vi "Login.vi"(8 "error in (no error)":errorcluster) -> (0 "error out":errorcluster)   [LabVIEW 2017]
uses:
  <vilib>/Utility/error.llb/DialogType.ctl
  Control/Login Authority CSV FGV Command.ctl
  Global/Login Details.vi
  Global/Global 1.vi
panel:
  in  "CANCEL":bool
  in  "LOGIN":bool
  in  "PASSWORD":string
  in  "USER NAME":string(combo)
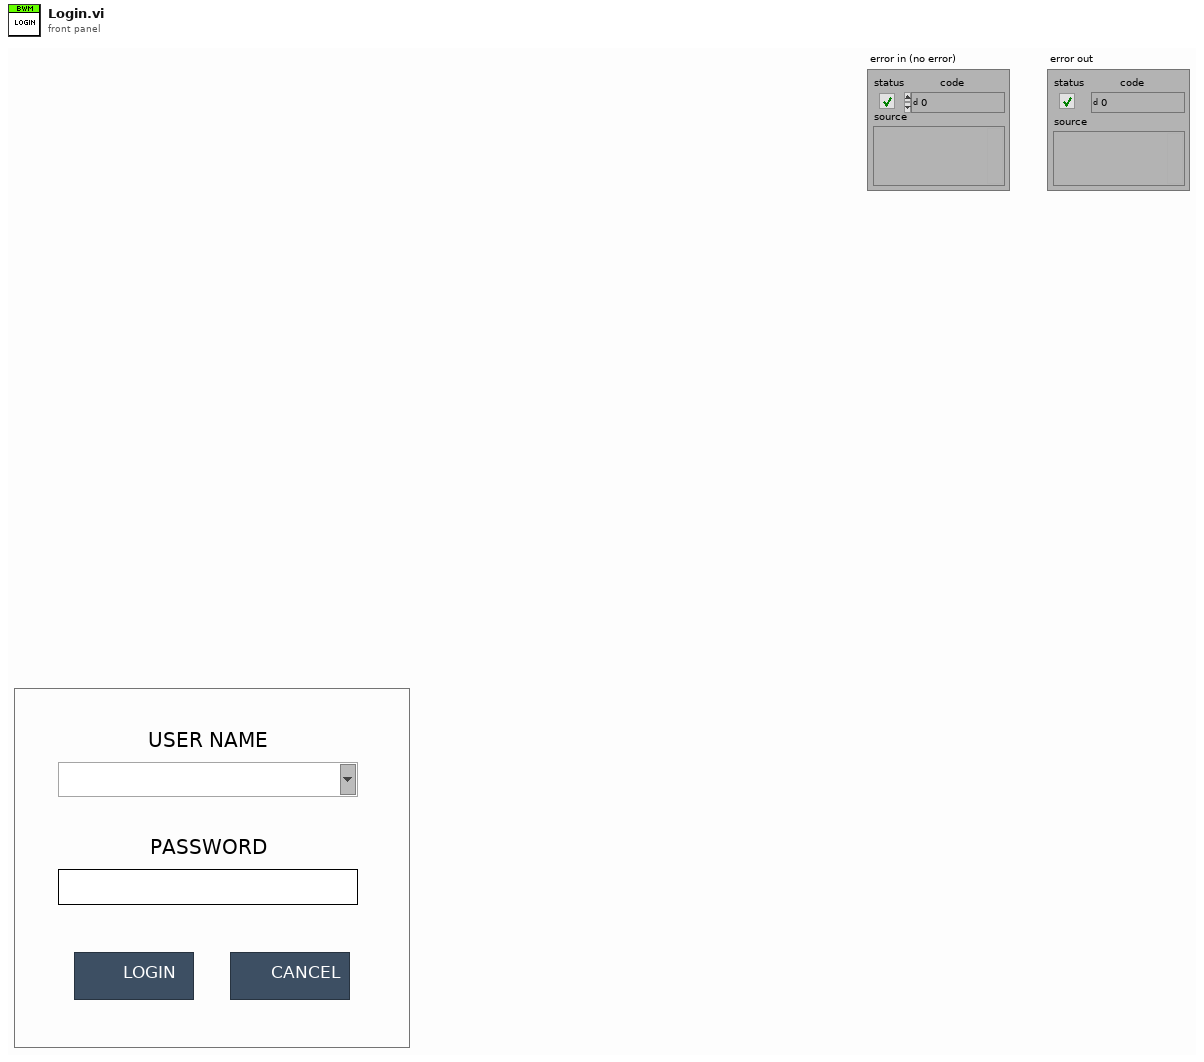
[diagram p1: front panel]
types:
  T1 = typedef "Login Authority CSV FGV Command.ctl" = enum16{"Init", "Save", "Read", "Get Data", "Delete"}
  T2 = typedef "DialogType.ctl" = u16
  T3 = enum32{"invalid app kind", "Development System", "Run Time System", "Student Edition", "Embedded LabVIEW", "Evaluation", "Custom"}
  T4 = cluster{"SCREEN 1":bool, "SCREEN 2":bool, "SCREEN 3":bool, "SCREEN 4":bool, "SCREEN 5":bool, "SCREEN 6":bool, "SCREEN 7":bool, "SCREEN 8":bool, "SCREEN 9":bool, "SCREEN 10":bool, "SCREEN 11":bool, "SCREEN 12":bool, "SCREEN 13":bool, "SCREEN 14":bool, "SCREEN 15":bool, "SCREEN 16":bool, "SCREEN 17":bool, "SCREEN 18":bool, "SCREEN 19":bool, "SCREEN 20":bool}
  T5 = cluster{"USERNAME":string, "AUTHORITY":string, "PASSWORD":string, "RE-ENTER PASSWORD":string}
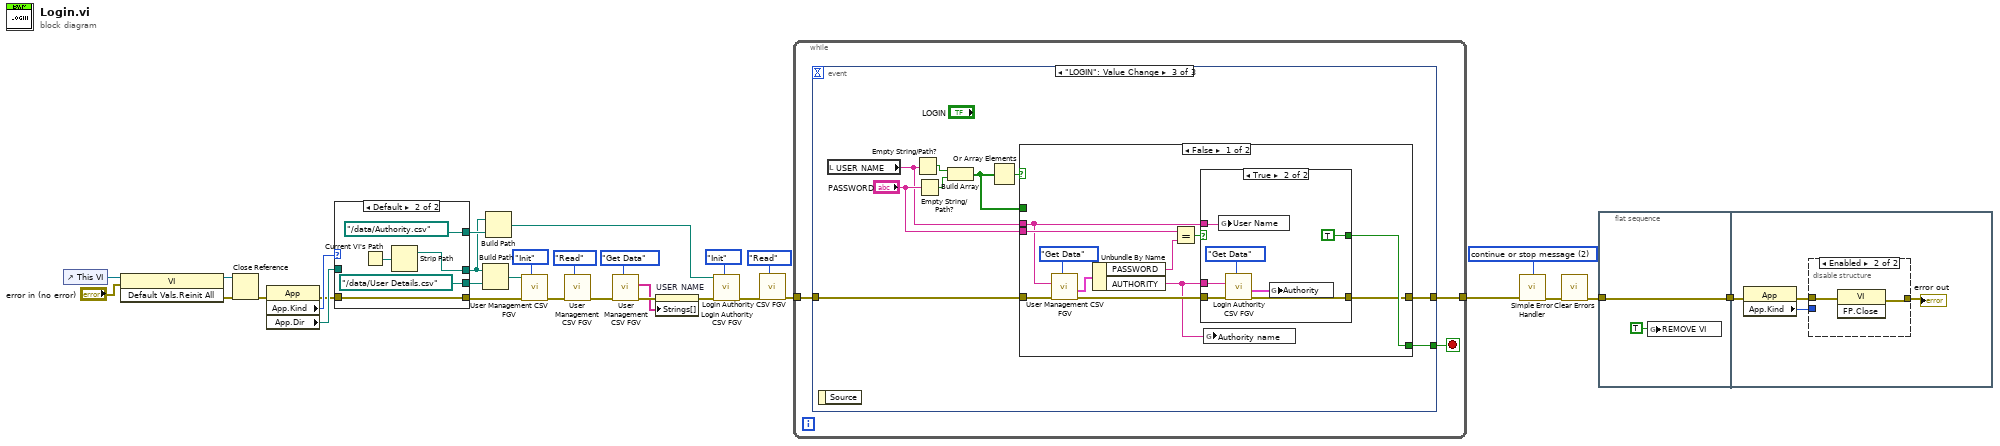
[diagram p0: block diagram]
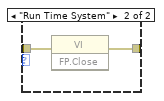
[diagram p3: hidden frame]
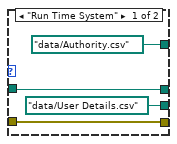
[diagram p4: hidden frame]
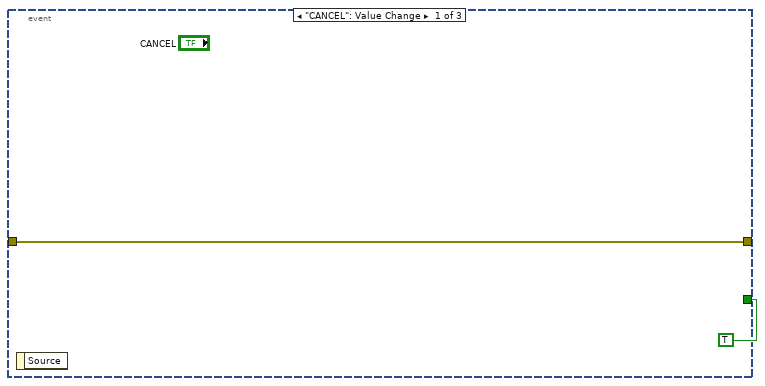
[diagram p5: hidden frame]
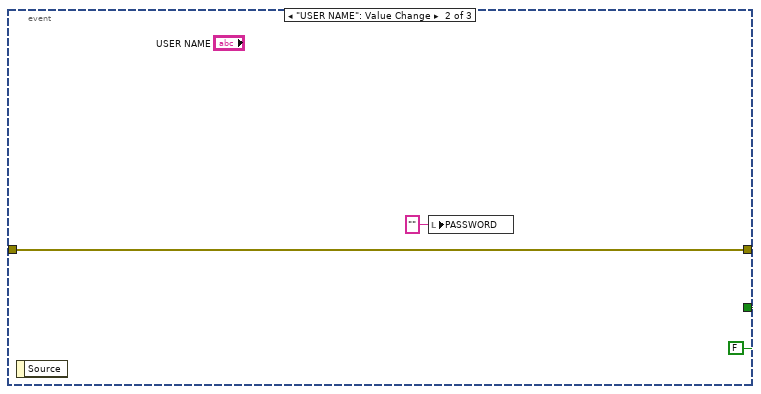
[diagram p6: hidden frame]
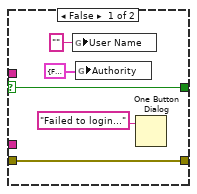
[diagram p7: hidden frame]
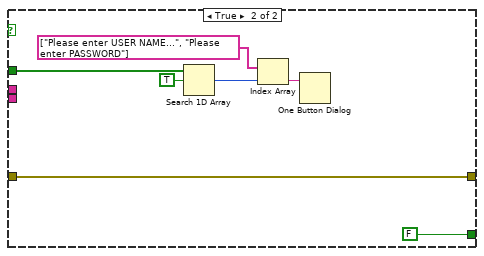
[diagram p8: hidden frame]
diagram:
  w20 = T2 2 items=["no dialog", "OK message", "continue or stop message", "OK message + warnings", "continue/stop + warnings"] ("type of dialog (OK msg:1)")
  n1 = control-ref of="This VI"() -> (w31:refnum<vi>)
  n2 = invoke class="VI" method="Default Vals.Reinit All"(reference=w31, error in="error in (no error)") -> (reference out=w28:refnum<vi>, error out=w29:errorcluster)  [unwired: 1 in, 1 out]
  n3 = Close Reference(reference=w28, error in (no error)=w29) -> (error out=w25:errorcluster)
  n4 = property class="App"(error in=w25) -> (error out=w24:errorcluster, "App.Kind"=w27:T3, "App.Dir"=w26:path)  [unwired: 1 in, 1 out]
  n5 = case shown="Default" w27 {
    tunnel: w26 -> [w35 _]
    tunnel: [path "data/User Details.csv" ("path") path "../data/User Details.csv" ("path")] -> w23
    tunnel: [w35 w38] -> w8
    tunnel: w24 -> [w33 w37]
    tunnel: [w33 w37] -> w11
    tunnel: [path "data/Authority.csv" ("path") path "../data/Authority.csv" ("path")] -> w9
    frame "Run Time System" {
    }
    frame Default {
      n6 = Current VI's Path() -> (path=w39:path)
      n7 = Strip Path(path=w39) -> (stripped path=w38:path)  [unwired: 1 out]
    }
  }
  n8 = Build Path(base path=w8, name or relative path=w23) -> (appended path=w10:path)
  n9 = Build Path(base path=w8, name or relative path=w9) -> (appended path=w2:path)
  n10 = call "User Management CSV FGV.vi"("Command"=Login_Authority_CSV_FGV_Command."Init", "error in (no error)"=w11, "Path"=w10) -> ("error out"=w18:errorcluster)  [unwired: 6 in, 2 out]
  n11 = call "User Management CSV FGV.vi"("Command"=Login_Authority_CSV_FGV_Command."Read", "error in (no error)"=w18) -> ("error out"=w17:errorcluster)  [unwired: 7 in, 2 out]
  n12 = call "User Management CSV FGV.vi"("Command"=Login_Authority_CSV_FGV_Command."Get Data", "error in (no error)"=w17) -> ("error out"=w13:errorcluster, "Usernames"=w12:string[])  [unwired: 7 in, 1 out]
  n13 = property on="USER NAME" class="CmbBox"(error in=w13, "Strings[]"=w12) -> (error out=w7:errorcluster)  [unwired: 1 in, 1 out]
  n14 = call "Login Authority CSV FGV.vi"("Command"=Login_Authority_CSV_FGV_Command."Init", "error in (no error)"=w7, "Path"=w2) -> ("error out"=w6:errorcluster)  [unwired: 6 in, 2 out]
  n15 = call "Login Authority CSV FGV.vi"("Command"=Login_Authority_CSV_FGV_Command."Read", "error in (no error)"=w6) -> ("error out"=w5:errorcluster)  [unwired: 7 in, 2 out]
  n16 = while {
    tunnel: w5 -> [w43]
    tunnel: [w42] -> w19
    stop <- w41 stop-if-true
    n17 = event shown="[2] \"LOGIN\": Value Change" {
      selector: _ -> [_ _ _]
      dyn-events: _ -> [_ _ _]
      timeout: _ -> [_ _ _]
      tunnel: w43 -> [w45 w47 w54]
      tunnel: [w45 w47 w55] -> w42
      tunnel: [TRUE FALSE w51] -> w41
      event "CANCEL": Value Change {
        n18 = event-data() -> ()  [unwired: 1 in, 1 out]
      }
      event "USER NAME": Value Change {
        n19 = event-data() -> ()  [unwired: 1 in, 1 out]
        n20 = local write "PASSWORD"("" ("PASSWORD")) -> ()
      }
      event "LOGIN": Value Change {
        n21 = event-data() -> ()  [unwired: 1 in, 1 out]
        n22 = local read "USER NAME"() -> (w49:string)
        n23 = Empty String/Path?(string/path=w49) -> (empty?=w57:bool)
        n24 = Empty String/Path?(string/path="PASSWORD") -> (empty?=w56:bool)
        n25 = Build Array(w57, w56) -> (w50:bool[])
        n26 = Or Array Elements(Boolean array=w50) -> (logical OR=w53:bool)
        n27 = case shown="False" w53 {
          tunnel: [w60 w87] -> w55
          tunnel: w54 -> [w66 w87]
          tunnel: w49 -> [w59 _]
          tunnel: "PASSWORD" -> [w64 _]
          tunnel: [w61 FALSE] -> w51
          tunnel: w50 -> [_ w85]
          frame False {
            n28 = call "User Management CSV FGV.vi"("Command"=Login_Authority_CSV_FGV_Command."Get Data", "error in (no error)"=w66, "Username"=w59) -> ("error out"=w62:errorcluster, "User data Out"=w67:T5)  [unwired: 6 in, 1 out]
            n29 = Unbundle By Name(w67) -> ("PASSWORD"=w65:string, "AUTHORITY"=w58:string)
            n30 = Equal?(x=w64, y=w65) -> (x = y?=w63:bool)
            n31 = case shown="True" w63 {
              selector: w63 -> [w73 _]
              tunnel: [w73 TRUE] -> w61
              tunnel: w62 -> [w72 w79]
              tunnel: [w72 w78] -> w60
              tunnel: w58 -> [_ w77]
              tunnel: w59 -> [_ w75]
              frame False {
                n32 = global write "Login Details.vi" "User Name"("" ("User Name")) -> ()
                n33 = global write "Login Details.vi" "Authority"(T4 {"SCREEN 1"=FALSE, "SCREEN 2"=FALSE, "SCREEN 3"=FALSE, "SCREEN 4"=FALSE, "SCREEN 5"=FALSE, "SCREEN 6"=FALSE, "SCREEN 7"=FALSE, "SCREEN 8"=FALSE, "SCREEN 9"=FALSE, "SCREEN 10"=FALSE, "SCREEN 11"=FALSE, "SCREEN 12"=FALSE, "SCREEN 13"=FALSE, "SCREEN 14"=FALSE, "SCREEN 15"=FALSE, "SCREEN 16"=FALSE, "SCREEN 17"=FALSE, "SCREEN 18"=FALSE, "SCREEN 19"=FALSE, "SCREEN 20"=FALSE} ("Authority")) -> ()
                n34 = One Button Dialog(message="Failed to login...") -> ()  [unwired: 1 in, 1 out]
              }
              frame True {
                n35 = global write "Login Details.vi" "User Name"(w75) -> ()
                n36 = call "Login Authority CSV FGV.vi"("Command"=Login_Authority_CSV_FGV_Command."Get Data", "error in (no error)"=w79, "Authority"=w77) -> ("error out"=w78:errorcluster, "Data Out"=w76:T4)  [unwired: 6 in, 1 out]
                n37 = global write "Login Details.vi" "Authority"(w76) -> ()
              }
            }
            n38 = global write "Login Details.vi" "Authority name"(w58) -> ()
          }
          frame True {
            n39 = Search 1D Array(1D array=w85, element=TRUE) -> (index of element=w83:i32)  [unwired: 1 in]
            n40 = Index Array(array=string[] ["Please enter USER NAME...", "Please enter PASSWORD"], index=w83) -> (element=w81:string)
            n41 = One Button Dialog(message=w81) -> ()  [unwired: 1 in, 1 out]
          }
        }
      }
    }
  }
  n42 = call <vilib>:"Simple Error Handler.vi"("type of dialog (OK msg:1)"=w20, "error in (no error)"=w19) -> ("error out"=w22:errorcluster)  [unwired: 3 in, 4 out]
  n43 = call <vilib>:"Clear Errors.vi"("error in (no error)"=w22) -> ("error out"=w21:errorcluster)  [unwired: 5 in, 1 out]
  n44 = flat-sequence {
    tunnel: w21 -> [w89]
    tunnel: [w89] -> w1
    tunnel: w1 -> [w91]
    frame #0 {
      n45 = global write "Global 1.vi" "REMOVE VI"(TRUE ("remove_VI")) -> ()
    }
    frame #1 {
      n46 = property class="App"(error in=w91) -> (error out=w92:errorcluster, "App.Kind"=w93:T3)  [unwired: 1 in, 1 out]
      n47 = disable-structure shown="Enabled" {
        disable-tunnel: w93 -> [w96 _]
        disable-tunnel: w92 -> [w95 w101]
        disable-tunnel: [w94 w100] -> w90
        frame Disabled {
          n48 = case shown="Default" w96 {
            tunnel: w95 -> [w97 w99]
            tunnel: [w97 w98] -> w94
            frame Default {
            }
            frame "Run Time System" {
              n49 = invoke class="VI" method="FP.Close"(error in=w99) -> (error out=w98:errorcluster)  [unwired: 2 in, 2 out]
            }
          }
        }
        frame Enabled {
          n50 = invoke class="VI" method="FP.Close"(error in=w101) -> (error out=w100:errorcluster)  [unwired: 2 in, 2 out]
        }
      }
      "error out" <- w90
    }
  }
